vi "_013.vi"() -> ()   [LabVIEW 2024]
panel:
  out "odd":dbl[](array[numeric])
  out "even":dbl[](array[numeric])
  # "Separating odd & even no's :"
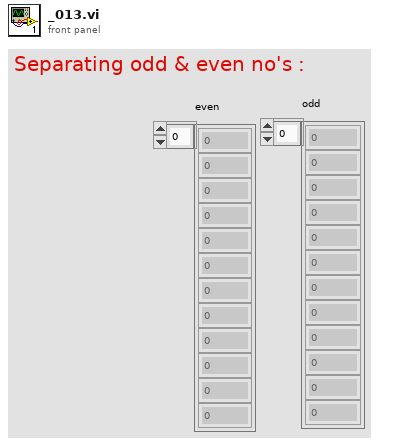
[diagram p1: front panel]
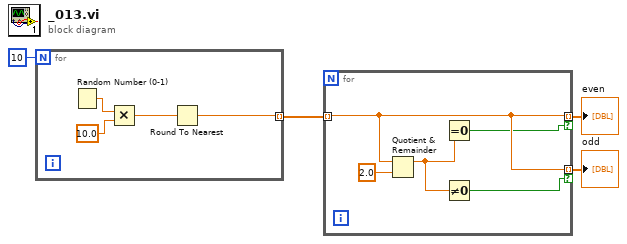
[diagram p0: block diagram]
diagram:
  n1 = for {
    N: 10 -> [_]
    tunnel: [w5] -> w3 mode=indexing
    n2 = Random Number (0-1)() -> (number: 0 to 1=w8:dbl)
    n3 = Multiply(x=w8, y=10.0) -> (x*y=w6:dbl)
    n4 = Round To Nearest(number=w6) -> (nearest integer value=w5:dbl)
  }
  n5 = for {
    tunnel: [w13] -> w2 mode=indexing if=w11
    tunnel: w3 -> [w13] mode=indexing
    tunnel: [w13] -> w1 mode=indexing if=w10
    n6 = Quotient & Remainder(x=w13, y=2.0) -> (x-y*floor(x/y)=w9:dbl)  [unwired: 1 out]
    n7 = Equal To 0?(x=w9) -> (x = 0?=w11:bool)
    n8 = Not Equal To 0?(x=w9) -> (x != 0?=w10:bool)
  }
  "even" <- w2
  "odd" <- w1
